vi "FPGA_controller.vi"() -> ()   [LabVIEW 2017]
uses:
  <vilib>/rvi/Emulation/niFpgaGetClockAttributes.vi
  <vilib>/rvi/Emulation/niFpgaSctlEmulationGetInTimedLoop.vi
  <vilib>/rvi/Emulation/niFpgaEmulationReportErrorSimple.vi
  <vilib>/rvi/eio/common/nirviEmuTemplateMethod_errors.vi
  <vilib>/rvi/Emulation/niFpgaCriticalErrorInLSC.vi
  <vilib>/eio/EIONode/EIONode.xnode
panel:
  out "Translated":i16
  out "VALID":bool
  in  "Scale x2":fxp<+/-,32,16>=10.0 format="%#_21g"
  in  "m_first x2":fxp<+/-,49,33>=4.9499969482421875 format="%#_26g"
  in  "Offset x2":fxp<+/-,48,32> format="%#_26g"
  in  "1/eta x":fxp<+/-,32,16>=200.0 format="%#_21g"
  in  "m_first x1":fxp<+/-,49,33>=0.649993896484375 format="%#_26g"
  in  "Offset x1":fxp<+/-,48,32> format="%#_26g"
  in  "Scale x1":fxp<+/-,32,16>=5.0 format="%#_21g"
  in  "stop":bool
  # "STATES CONVERSION"
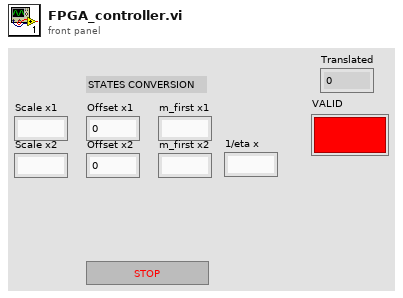
[diagram p1: front panel]
types:
  T1 = cluster{"Boolean array[0]":bool, "Boolean array[1]":bool, "Boolean array[2]":bool, "Boolean array[3]":bool, "Boolean array[4]":bool, "Boolean array[5]":bool, "Boolean array[6]":bool, "Boolean array[7]":bool, "Boolean array[8]":bool, "Boolean array[9]":bool, "Boolean array[10]":bool, "Boolean array[11]":bool, "Boolean array[12]":bool, "Boolean array[13]":bool, "Boolean array[14]":bool, "Boolean array[15]":bool}
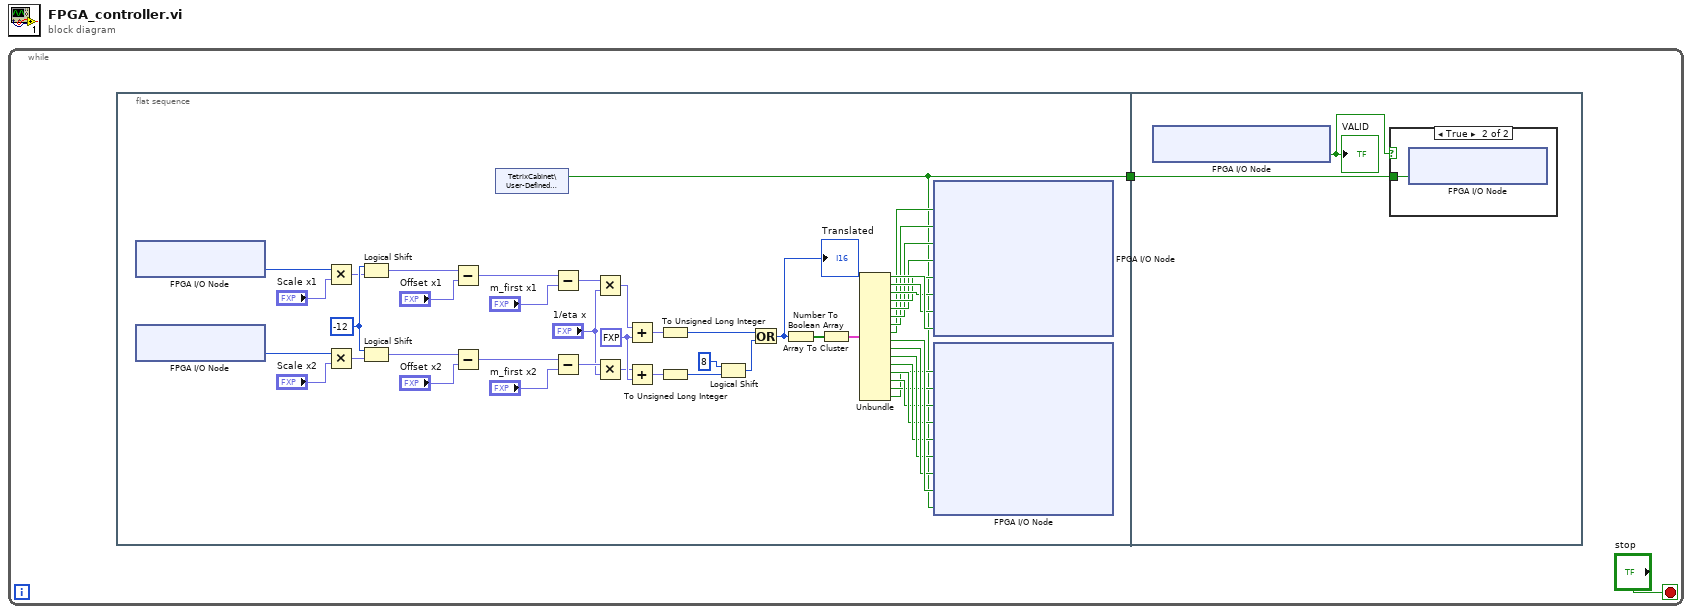
[diagram p0: block diagram]
diagram:
  n1 = while {
    stop <- "stop" stop-if-true
    n2 = flat-sequence {
      tunnel: [w3] -> w1
      tunnel: w1 -> [w51]
      frame #0 {
        w27 = fxp<+/-,64,32> 0.5 ("y")
        w25 = i16 -12 ("y")
        n3 = xnode "FPGA I/O Node"() -> ("ConnectorA/AI0"=w15:u16)  [unwired: 1 in, 1 out]
        n4 = xnode "FPGA I/O Node"() -> ("ConnectorA/AI1"=w14:u16)  [unwired: 1 in, 1 out]
        n5 = Multiply(x=w15, y="Scale x1") -> (x*y=w24:fxp<+/-,48,32>)
        n6 = Multiply(x=w14, y="Scale x2") -> (x*y=w28:fxp<+/-,48,32>)
        n7 = Logical Shift(y=w25, x=w24) -> (x << y=w21:fxp<+/-,48,32>)
        n8 = Logical Shift(y=w25, x=w28) -> (x << y=w18:fxp<+/-,48,32>)
        n9 = Subtract(x=w21, y="Offset x1") -> (x-y=w22:fxp<+/-,49,33>)
        n10 = Subtract(x=w18, y="Offset x2") -> (x-y=w19:fxp<+/-,49,33>)
        n11 = shared-variable "TetrixCabinet\\User-Defined Variables\\Input"() -> (w3:bool)  [unwired: 1 in, 1 out]
        n12 = Subtract(x=w22, y="m_first x1") -> (x-y=w23:fxp<+/-,50,34>)
        n13 = Subtract(x=w19, y="m_first x2") -> (x-y=w17:fxp<+/-,50,34>)
        n14 = Multiply(x=w23, y="1/eta x") -> (x*y=w20:fxp<+/-,64,49>)
        n15 = Multiply(x=w17, y="1/eta x") -> (x*y=w16:fxp<+/-,64,49>)
        n16 = Add(x=w20, y=w27) -> (x+y=w31:fxp<+/-,64,50>)
        n17 = Add(x=w16, y=w27) -> (x+y=w26:fxp<+/-,64,50>)
        n18 = To Unsigned Long Integer(number=w31) -> (unsigned 32bit integer=w6:u32)
        n19 = To Unsigned Long Integer(number=w26) -> (unsigned 32bit integer=w29:u32)
        n20 = Logical Shift(y=8, x=w29) -> (x << y=w5:u32)
        n21 = Or(x=w6, y=w5) -> (x .or. y?=w4:u32)
        "Translated" <- w4
        n22 = Number To Boolean Array(number=w4) -> (Boolean array=w48:bool[])
        n23 = Array To Cluster(array=w48) -> (cluster=w49:T1)
        n24 = Unbundle(w49) -> ("Boolean array[0]"=w47:bool, "Boolean array[1]"=w46:bool, "Boolean array[2]"=w45:bool, "Boolean array[3]"=w44:bool, "Boolean array[4]"=w43:bool, "Boolean array[5]"=w42:bool, "Boolean array[6]"=w41:bool, "Boolean array[7]"=w40:bool, "Boolean array[8]"=w39:bool, "Boolean array[9]"=w38:bool, "Boolean array[10]"=w37:bool, "Boolean array[11]"=w36:bool, "Boolean array[12]"=w35:bool, "Boolean array[13]"=w34:bool, "Boolean array[14]"=w33:bool, "Boolean array[15]"=w32:bool)
        n25 = xnode "FPGA I/O Node"("Component-Level IP\\pi00"=w40, "Component-Level IP\\pi01"=w41, "Component-Level IP\\pi02"=w42, "Component-Level IP\\pi03"=w43, "Component-Level IP\\pi04"=w44, "Component-Level IP\\pi05"=w45, "Component-Level IP\\pi06"=w46, "Component-Level IP\\pi07"=w47) -> ()  [unwired: 8 in, 8 out]
        n26 = xnode "FPGA I/O Node"("Component-Level IP\\pi08"=w32, "Component-Level IP\\pi09"=w33, "Component-Level IP\\pi10"=w34, "Component-Level IP\\pi11"=w35, "Component-Level IP\\pi12"=w36, "Component-Level IP\\pi13"=w37, "Component-Level IP\\pi14"=w38, "Component-Level IP\\pi15"=w39, "Component-Level IP\\pi16"=w3) -> ()  [unwired: 9 in, 9 out]
      }
      frame #1 {
        n27 = xnode "FPGA I/O Node"() -> ("Component-Level IP\\po0"=w50:bool)  [unwired: 1 in, 1 out]
        "VALID" <- w50
        n28 = case shown="True" w50 {
          tunnel: w51 -> [_ w52]
          frame False {
          }
          frame True {
            n29 = xnode "FPGA I/O Node"("ConnectorA/DIO0"=w52) -> ()  [unwired: 1 in, 1 out]
          }
        }
      }
    }
  }
